vi "Append Asset Metadata.vi"(4 "Value":string, 6 "Property":string, 8 "error in (no error)":errorcluster, 10 "Properties":string[][](array[string]), 11 "Asset ID":string) -> (0 "error out":errorcluster)   [LabVIEW 2024]
uses:
  SupportVIs/Header--Combo Box.ctl
  SupportVIs/Format JSON Object.vi
  SupportVIs/PATCH (Buffer).vi
  SupportVIs/Session.lvclass
  SupportVIs/NI Skyline Configuration Library.lvlib
  SupportVIs/JSONtext.lvlib
panel:
  out "buffer":string
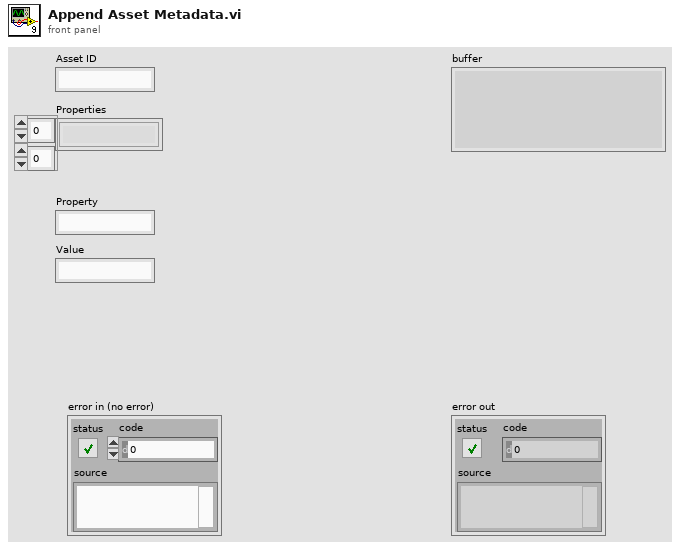
[diagram p1: front panel]
types:
  T1 = typedef "lib_NI_Advanced HTTP Client.lvlib/Session.lvclass/Header--Combo Box.ctl" = string
  T2 = typedef "NI Skyline Configuration Library.lvlib/Auto Configuration.ctl" = cluster{"id":string, "uri":string, "api key":string, "cert path":path, "owning file":path}
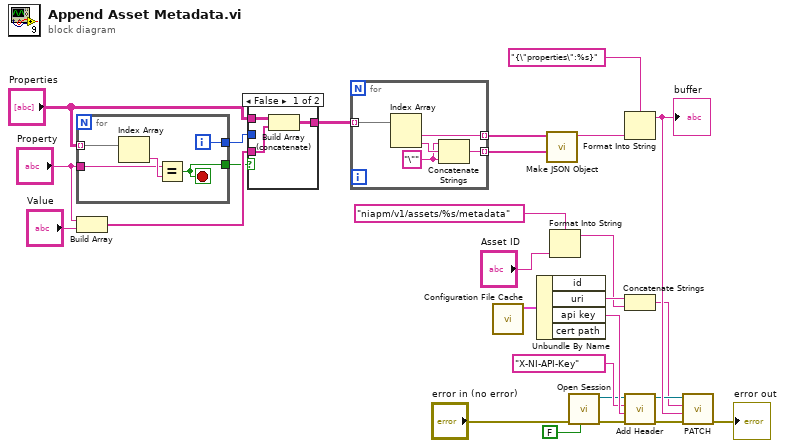
[diagram p0: block diagram]
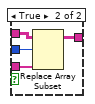
[diagram p2: hidden frame]
diagram:
  n1 = for {
    tunnel: "Properties" -> [w32] mode=indexing
    tunnel: "Property" -> [w30]
    tunnel: [w29] -> w20
    tunnel: [w28] -> w16
    i -> [w28]
    stop <- w29 stop-if-true
    n2 = Index Array(array=w32) -> (element=w31:string)  [unwired: 1 in]
    n3 = Equal?(x=w30, y=w31) -> (x = y?=w29:bool)
  }
  n4 = Build Array("Property", "Value") -> (w21:string[])
  n5 = case shown="False" w20 {
    tunnel: w16 -> [_ w39]
    tunnel: "Properties" -> [w35 w38]
    tunnel: w21 -> [w34 w37]
    tunnel: [w33 w36] -> w22
    frame False {
      n6 = Build Array (concatenate)(w35, w34) -> (w33:string[][])
    }
    frame True {
      n7 = Replace Array Subset(array=w38, new element=w37, index (row)=w39) -> (w36:string[][])  [unwired: 1 in]
    }
  }
  n8 = for {
    tunnel: w22 -> [w44] mode=indexing
    tunnel: [w43] -> w23 mode=indexing
    tunnel: [w41] -> w27 mode=indexing
    w40 = "\"" ("string")
    n9 = Index Array(array=w44) -> (element #1=w43:string, element #2=w42:string)  [unwired: 2 in]
    n10 = Concatenate Strings(w40, w42, w40) -> (w41:string)
  }
  n11 = call "Configuration File Cache.vi"() -> ("HTTP configuration"=w7:T2)  [unwired: 10 in, 1 out]
  n12 = Unbundle By Name(w7) -> ("uri"=w14:string, "api key"=w13:string)  [unwired: 2 out]
  n13 = call "Make JSON Object.vi"("JSON Items"=w27, "Item Names"=w23) -> ("<JSON>"=w25:string)  [unwired: 8 in, 1 out]
  n14 = Format Into String(format string="niapm/v1/assets/%s/metadata" ("url"), "Asset ID") -> (resulting string=w2:string)  [unwired: 2 in, 1 out]
  n15 = call "Open Session.vi"("verify server (T)"=FALSE, "error in"="error in (no error)") -> ("error out"=w11:errorcluster, "session"=w8:refnum<class "Session.lvclass">)  [unwired: 8 in]
  n16 = Format Into String(format string="{\"properties\":%s}" ("JSON"), w25) -> (resulting string=w26:string)  [unwired: 2 in, 1 out]
  "buffer" <- w26
  n17 = Concatenate Strings(w14, w2) -> (w4:string)
  n18 = call "Add Header.vi"("error in"=w11, "value"=w13, "header"=T1 "X-NI-API-Key", "session in"=w8) -> ("error out"=w10:errorcluster, "session out"=w9:refnum<class "Session.lvclass">)  [unwired: 6 in]
  n19 = call-poly "PATCH.vi"("error in"=w10, "buffer"=w26, "url"=w4, "session in"=w9) -> ("error out"=→"error out":errorcluster)  [unwired: 3 in, 4 out]
